vi "Read Position.vi"(9 "GObject in":refnum<class "GObject.lvclass">) -> (3 "GObject out":refnum<class "GObject.lvclass">, 4 "Position":T1)   [LabVIEW 2014, in "Raspberry Pi Compatible Compiler for LabVIEW.lvlib" / "GObject.lvclass"]
uses:
  GObject.lvclass
  <vilib>/Utility/miscctls.llb/LVPositionTypeDef.ctl
  GObject.lvclass/GObject.ctl
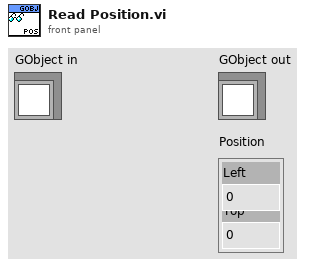
[diagram p1: front panel]
types:
  T1 = typedef "LVPositionTypeDef.ctl" = cluster{"Left":i32, "Top":i32}
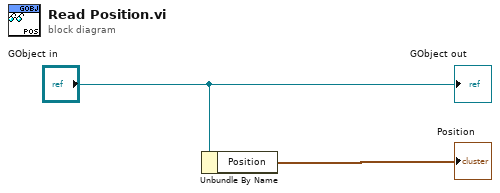
[diagram p0: block diagram]
diagram:
  n1 = Unbundle By Name("GObject in") -> ("Position"=→"Position":T1)
  "GObject out" <- "GObject in"
